vi "ellipse parameter estimate.vi"(10 "Y":dbl[](array[numeric]), 11 "X":dbl[](array[numeric])) -> (0 "y0":dbl, 1 "x0":dbl, 2 "b":dbl, 3 "a":dbl)   [LabVIEW 2023]
doc: "Ellipse parameter estimate"
uses:
  <vilib>/gmath/NI_Gmath.lvlib
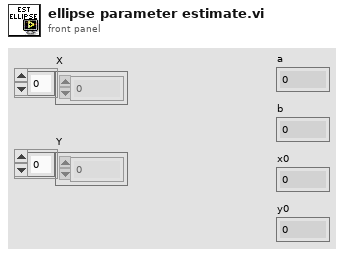
[diagram p1: front panel]
types:
  T1 = enum16{"arithmetic", "geometric", "harmonic", "trimmed", "median"}
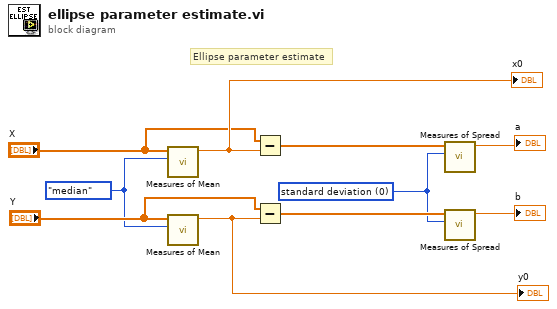
[diagram p0: block diagram]
diagram:
  w3 = 0 items=["standard deviation", "range", "mean absolute deviation", "interquartile range"] ("type")
  w9 = T1."median" ("type")
  # "Ellipse parameter estimate"
  n1 = call <vilib>:"Measures of Mean.vi"("type"=w9, "x array"="X") -> ("mean value"=w8:dbl)  [unwired: 8 in, 1 out]
  "x0" <- w8
  n2 = call <vilib>:"Measures of Mean.vi"("type"=w9, "x array"="Y") -> ("mean value"=w7:dbl)  [unwired: 8 in, 1 out]
  "y0" <- w7
  n3 = Subtract(x="X", y=w8) -> (x-y=w5:dbl[])
  n4 = Subtract(x="Y", y=w7) -> (x-y=w4:dbl[])
  n5 = call <vilib>:"Measures of Spread.vi"("type"=w3, "x array"=w5) -> ("spread value"=→"a":dbl)  [unwired: 8 in, 1 out]
  n6 = call <vilib>:"Measures of Spread.vi"("type"=w3, "x array"=w4) -> ("spread value"=→"b":dbl)  [unwired: 8 in, 1 out]
